vi "Set Scale.vi"(8 "error in (no error)":errorcluster, 10 "Scale":cluster{"X":sgl, "Y":sgl, "Z":sgl}, 11 "Scene Object":refnum<vi>) -> (0 "error out":errorcluster, 3 "Scaled Object":refnum<vi>)   [LabVIEW 2020, in "NI_3D Picture Control.lvlib"]
doc: "Clears any previous scale operation applied to an object in a 3D scene and applies the scaling factors you specify. This VI performs an absolute scale from the object's initial position."
uses:
  <vilib>/picture/3D Picture Control/NI_3D Picture Control.lvlib
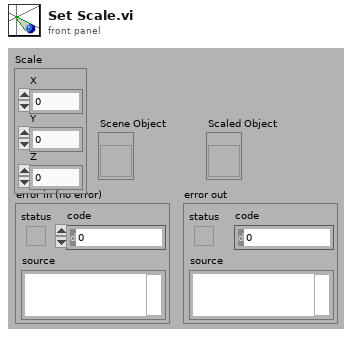
[diagram p1: front panel]
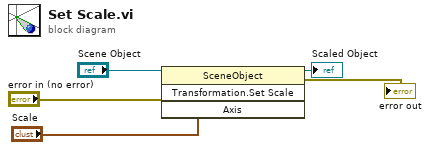
[diagram p0: block diagram]
diagram:
  n1 = invoke class="SceneObject" method="Transformation.Set Scale"(reference="Scene Object", error in="error in (no error)", "Axis"="Scale") -> (reference out=→"Scaled Object":refnum<vi>, error out=→"error out":errorcluster)  [unwired: 1 in, 2 out]
